vi "AlliGator Check Version.vi"   [LabVIEW 2021, in "AlliGator GUI.lvlib"]
doc: "Compares the current AlliGator version to the latest released one on Github.\nIf a newer version is available, offers to download and install it."
uses:
  AlliGator GUI.lvlib
  Globals, Variables, Constants/AlliGator Globals.vi
  Globals, Variables, Constants/AlliGator Globals, Variables & Constants.lvlib
  Error/Error.lvlib
panel:
  # "see the AlliGator License on the block diagram (Ctrl+E or Window:Show Block Diagram)"
types:
  T1 = enum16{"Left Button", "Center Button", "Right Button", "Window Close"}
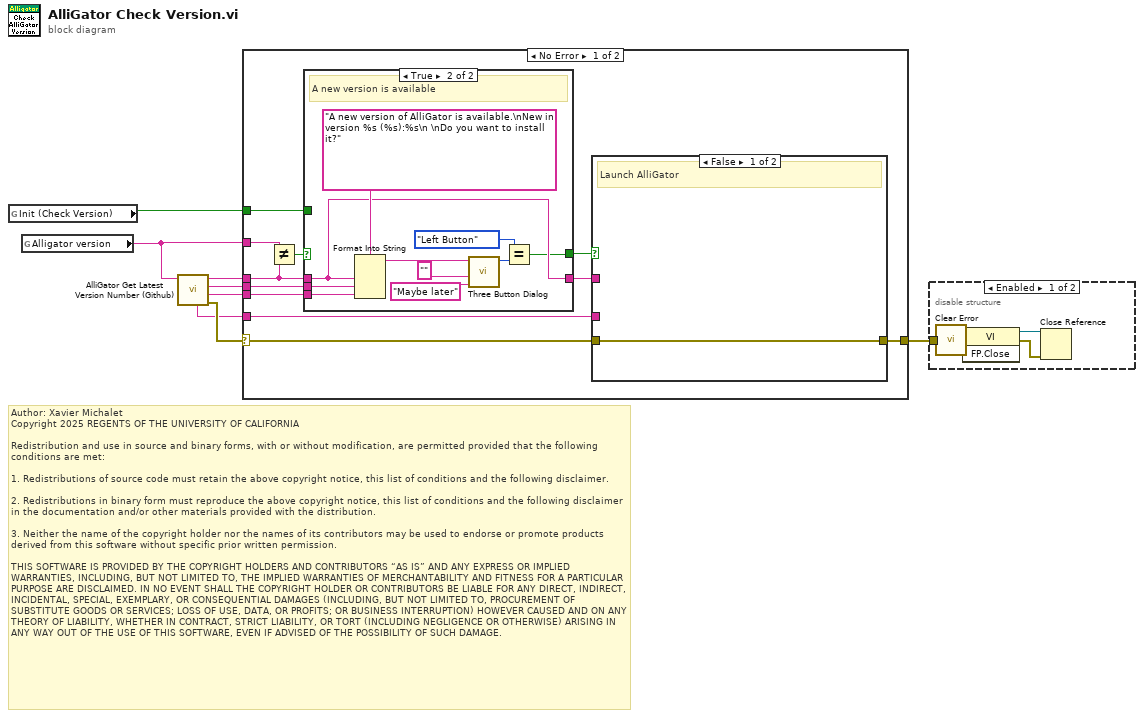
[diagram p0: block diagram]
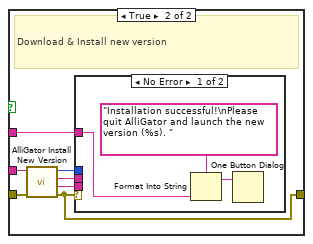
[diagram p2: hidden frame]
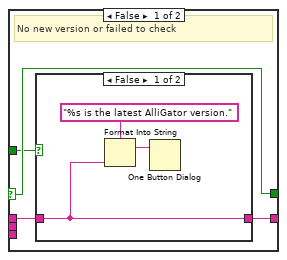
[diagram p4: hidden frame]
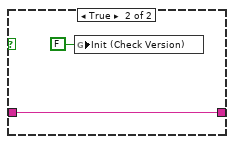
[diagram p5: hidden frame]
diagram:
  # "Author: Xavier Michalet\nCopyright 2025 REGENTS OF THE UNIVERSITY OF CALIFORNIA\n\nRedistribution and use in source and binary forms, with or without modification, are permitted provided that the following conditions are met:\n\n1. Redistributions of source code must retain the above copyright notice, this list of conditions and the following disclaimer.\n\n2. Redistributions in binary form must reproduce the above copyright notice, this list of conditions and the following disclaimer in the documentation and/or other materials provided with the distribution.\n\n3. Neither the name of the copyright holder nor the names of its contributors may be used to endorse or promote products derived from this software without specific prior written permission.\n\nTHIS SOFTWARE IS PROVIDED BY THE COPYRIGHT HOLDERS AND CONTRIBUTORS “AS IS” AND ANY EXPRESS OR IMPLIED WARRANTIES, INCLUDING, BUT NOT LIMITED TO, THE IMPLIED WARRANTIES OF MERCHANTABILITY AND FITNESS FOR A PARTICULAR PURPOSE ARE DISCLAIMED. IN NO EVENT SHALL THE COPYRIGHT HOLDER OR CONTRIBUTORS BE LIABLE FOR ANY DIRECT, INDIRECT, INCIDENTAL, SPECIAL, EXEMPLARY, OR CONSEQUENTIAL DAMAGES (INCLUDING, BUT NOT LIMITED TO, PROCUREMENT OF SUBSTITUTE GOODS OR SERVICES; LOSS OF USE, DATA, OR PROFITS; OR BUSINESS INTERRUPTION) HOWEVER CAUSED AND ON ANY THEORY OF LIABILITY, WHETHER IN CONTRACT, STRICT LIABILITY, OR TORT (INCLUDING NEGLIGENCE OR OTHERWISE) ARISING IN ANY WAY OUT OF THE USE OF THIS SOFTWARE, EVEN IF ADVISED OF THE POSSIBILITY OF SUCH DAMAGE."
  n1 = global read "AlliGator Globals.vi" "Init (Check Version)"() -> (w4:bool)
  n2 = global read "AlliGator Globals.vi" "Alligator version"() -> (w5:string)
  n3 = call "AlliGator Get Latest Version Number (Github).vi"("Current Version"=w5) -> ("Error Out"=w7:errorcluster, "New in this Version"=w2:string, "Release Date"=w3:string, "Latest Version"=w8:string, "Latest Version Installer Web Address"=w1:string)  [unwired: 6 in]
  n4 = case shown="No Error" w7 {
    selector: w7 -> [w17 w50]
    tunnel: w8 -> [w18 _]
    tunnel: [w15 w50] -> w6
    tunnel: w5 -> [w14 _]
    tunnel: w4 -> [w13 _]
    tunnel: w3 -> [w11 _]
    tunnel: w2 -> [w10 _]
    tunnel: w1 -> [w9 _]
    frame No Error {
      n5 = Not Equal?(x=w14, y=w18) -> (x != y?=w19:bool)
      n6 = case shown="True" w19 {
        selector: w19 -> [w34 _]
        tunnel: w18 -> [w33 w48]
        tunnel: [w34 w40] -> w16
        tunnel: w11 -> [_ w47]
        tunnel: w13 -> [w32 _]
        tunnel: [w31 w48] -> w12
        tunnel: w10 -> [_ w46]
        frame False {
          # "No new version or failed to check"
          n7 = case shown="False" w32 {
            tunnel: w33 -> [w35 w38]
            tunnel: [w35 w38] -> w31
            frame False {
              n8 = Format Into String(format string="%s is the latest AlliGator version." ("message"), w35) -> (resulting string=w37:string)  [unwired: 2 in, 1 out]
              n9 = One Button Dialog(message=w37) -> ()  [unwired: 1 in, 1 out]
            }
            frame True {
              n10 = global write "AlliGator Globals.vi" "Init (Check Version)"(FALSE ("Init (Check Version)")) -> ()
            }
          }
        }
        frame True {
          # "A new version is available"
          n11 = Format Into String(format string="A new version of AlliGator is available.\nNew in version %s (%s):%s\n \nDo you want to install it?" ("message"), w48, w47, w46) -> (resulting string=w45:string)  [unwired: 2 in, 1 out]
          n12 = call <vilib>:"Three Button Dialog.vi"("Right Button Text (\"Cancel\")"="Maybe later" ("F button name (\"Cancel\")"), "Center Button Text (\"No\")"="" ("Center Button Text (\"No\")"), "message"=w45) -> ("Which Button?"=w42:T1)  [unwired: 8 in]
          n13 = Equal?(x=T1."Left Button" ("Which Button?"), y=w42) -> (x = y?=w40:bool)
        }
      }
      n14 = case shown="False" w16 {
        tunnel: w9 -> [_ w27]
        tunnel: w17 -> [w20 w26]
        tunnel: [w20 w25] -> w15
        tunnel: w12 -> [_ w24]
        frame False {
          # "Launch AlliGator"
        }
        frame True {
          # "Download & Install new version"
          n15 = call "AlliGator Install New Version.vi"("Error In"=w26, "AlliGator Installer Web Address"=w27) -> ("Error Out"=w25:errorcluster, "standard error"=w21:string, "standard output"=w22:string, "return code"=w23:i32)  [unwired: 6 in]
          n16 = case shown="No Error" w25 {
            tunnel: w24 -> [w28 _]
            tunnel: w23 -> [_ _]
            tunnel: w22 -> [_ _]
            tunnel: w21 -> [_ _]
            frame No Error {
              n17 = Format Into String(format string="Installation successful!\nPlease quit AlliGator and launch the new version (%s). " ("message"), w28) -> (resulting string=w29:string)  [unwired: 2 in, 1 out]
              n18 = One Button Dialog(message=w29) -> ()  [unwired: 1 in, 1 out]
            }
            frame Error {
            }
          }
        }
      }
    }
    frame Error {
    }
  }
  n19 = disable-structure shown="Enabled" {
    disable-tunnel: w6 -> [w54 _]
    frame Enabled {
      n20 = call "Clear Error.vi"("Error In"=w54) -> ("no Error Out"=w53:errorcluster)  [unwired: 8 in]
      n21 = invoke class="VI" method="FP.Close"(error in=w53) -> (reference out=w52:refnum<vi>, error out=w51:errorcluster)  [unwired: 2 in, 1 out]
      n22 = Close Reference(reference=w52, error in (no error)=w51) -> ()  [unwired: 1 out]
    }
    frame Disabled {
    }
  }
